vi "CreateJSONFile.vi"() -> (2 "Path":path)   [LabVIEW 2018]
uses:
  Global Variables.vi
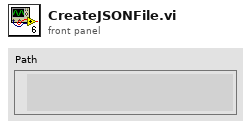
[diagram p1: front panel]
types:
  T1 = enum16{"open", "replace", "create", "open or create", "replace or create", "replace or create with confirmation"}
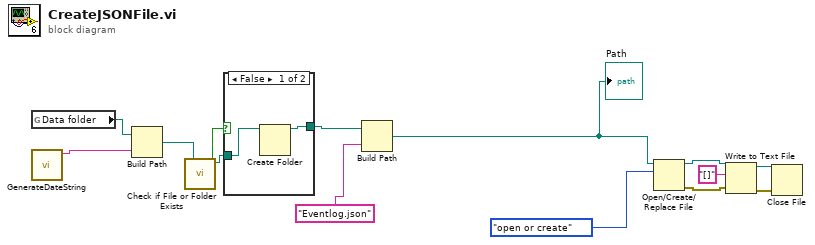
[diagram p0: block diagram]
diagram:
  n1 = global read "Global Variables.vi" "Data folder"() -> (w7:path)
  n2 = call "GenerateDateString.vi"() -> ("String"=w8:string)  [unwired: 11 in]
  n3 = Build Path(base path=w7, name or relative path=w8) -> (appended path=w11:path)
  n4 = call <vilib>:"Check if File or Folder Exists.vi"("path"=w11) -> ("file or folder exists?"=w9:bool, "dup path"=w10:path)  [unwired: 8 in, 1 out]
  n5 = case shown="False" w9 {
    tunnel: w10 -> [w16 w17]
    tunnel: [w15 w17] -> w12
    frame False {
      n6 = Create Folder(path (use dialog)=w16) -> (created path=w15:path)  [unwired: 2 in, 2 out]
    }
    frame True {
    }
  }
  n7 = Build Path(base path=w12, name or relative path="Eventlog.json" ("string")) -> (appended path=w6:path)
  "Path" <- w6
  n8 = Open/Create/Replace File(file path (use dialog)=w6, operation (0:open)=T1."open or create") -> (refnum out=w4:refnum<file>, error out=w3:errorcluster)  [unwired: 4 in, 1 out]
  n9 = Write to Text File(file (use dialog)=w4, text="[]", error in=w3) -> (refnum out=w1:refnum<file>, error out=w2:errorcluster)  [unwired: 1 in, 1 out]
  n10 = Close File(refnum=w1, error in=w2) -> ()  [unwired: 2 out]
